vi "Get Parents.vi"(8 "error in (no error)":errorcluster, 10 "ID":i32=-1, 11 "Parent Child in":refnum<class "Parent Child.lvclass">) -> (0 "error out":errorcluster, 1 "Parents":i32[](array[numeric]), 3 "Parent Child out":refnum<class "Parent Child.lvclass">)   [LabVIEW 2019, in "HierDAL Library.lvlib" / "Database.lvlib" / "Repositories.lvlib" / "Parent Child.lvclass"]
uses:
  Parent Child.lvclass
  Parent Child.lvclass/Parent Child.ctl
  Database Manager Class/Database Manager.lvclass
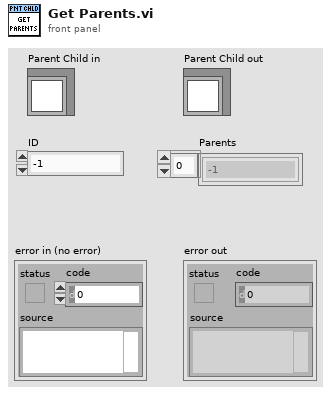
[diagram p1: front panel]
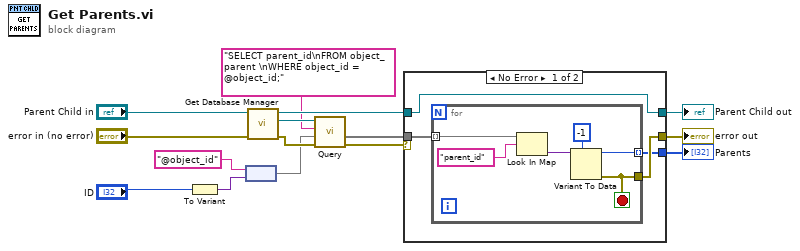
[diagram p0: block diagram]
diagram:
  n1 = To Variant(anything="ID") -> (Variant=w12:variant)
  n2 = node("@object_id" ("key"), w12) -> (w7:map{string, variant})
  n3 = call "Get Database Manager.vi"("error in (no error)"="error in (no error)", "Parent Child in"="Parent Child in") -> ("error out"=w8:errorcluster, "Database Manager"=w9:refnum<class "Database Manager.lvclass">, "Parent Child out"=w15:refnum<class "Parent Child.lvclass">)  [unwired: 7 in]
  n4 = call-dynamic "Query.vi"("error in (no error)"=w8, "Parameters"=w7, "Query"="SELECT parent_id\nFROM object_parent \nWHERE object_id = @object_id;", "Database Manager in"=w9) -> ("error out"=w5:errorcluster, "Rows"=w4:map{string, variant}[])  [unwired: 5 in, 1 out]
  n5 = case shown="No Error" w5 {
    selector: w5 -> [_ w26]
    tunnel: w4 -> [w18 _]
    tunnel: w15 -> [w19 w27]
    tunnel: [w19 w27] -> w3
    tunnel: [w17 w26] -> w2
    tunnel: [w16 _] -> w1
    frame No Error {
      n6 = for {
        tunnel: w18 -> [w24] mode=indexing
        tunnel: [w22] -> w16 mode=indexing
        tunnel: [w21] -> w17
        stop <- w21 stop-if-true
        n7 = Look In Map(map=w24, key="parent_id") -> (value=w25:variant)  [unwired: 1 in, 1 out]
        n8 = Variant To Data(type=-1 ("ID"), Variant=w25) -> (data=w22:i32, error out=w21:errorcluster)  [unwired: 1 in]
      }
    }
    frame Error {
    }
  }
  "error out" <- w2
  "Parent Child out" <- w3
  "Parents" <- w1
